vi "Get SMO Public API.vi"(8 "error in (no error)":errorcluster, 11 "Inst.Krohn-Hite-7008 in":refnum<class "Inst.Krohn-Hite-7008.lvclass">) -> (0 "error out":errorcluster, 2 "Commands":string[](array[string]), 3 "Inst.Krohn-Hite-7008 out":refnum<class "Inst.Krohn-Hite-7008.lvclass">)   [LabVIEW 2019, in "Inst.KH7008.lvlib" / "Inst.Krohn-Hite-7008.lvclass"]
uses:
  Inst.Krohn-Hite-7008.lvclass
  Typedefs/Inst.Krohn-Hite-7008.Commands--Enum.ctl
  d076ed97-22e4-4017-a7d1-2daba86b0ad5.vi
  5bb7ec78-ffd5-4b96-a1c9-711a63f6b5b1.vi
  <vilib>/Utility/Data Type/Get Type Information.vi
  <vilib>/Utility/Data Type/Get Numeric Information.vi
  <userlib>/_OpenG.lib/lvdata/lvdata.llb/Unwrap VVariant__ogtk.vi
  <userlib>/LevyLab/Instrument Framework/Instrument Types/Amplifier/Instrument.Amplifier.lvclass
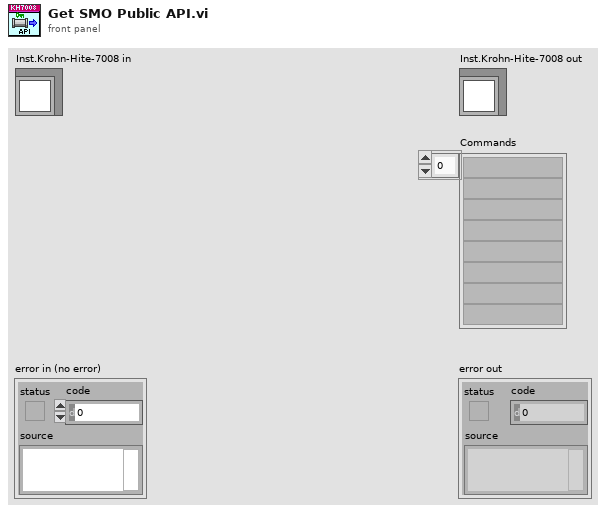
[diagram p1: front panel]
types:
  T1 = typedef "Inst.KH7008.lvlib/Inst.Krohn-Hite-7008.lvclass/Inst.Krohn-Hite-7008.Commands--Enum.ctl" = enum16{"getChannel", "getAllChannels", "setChannel", "setAllChannels"}
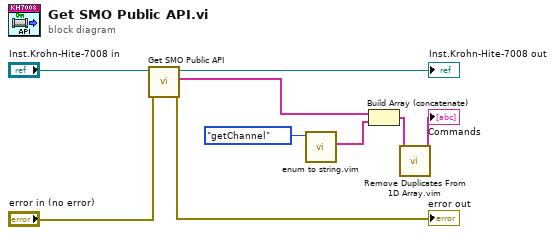
[diagram p0: block diagram]
diagram:
  n1 = call-parent "Get SMO Public API.vi"("error in (no error)"="error in (no error)", "Instrument.Amplifier in"="Inst.Krohn-Hite-7008 in") -> ("error out"=→"error out":errorcluster, "commands"=w9:string[], "Instrument.Amplifier out"=→"Inst.Krohn-Hite-7008 out":refnum<class "Inst.Krohn-Hite-7008.lvclass">)  [unwired: 7 in]
  n2 = call "enum to string.vim"("enum in"=Inst.Krohn-Hite-7008.Commands--Enum."getChannel" ("Commands")) -> ("strings out"=w5:string[])  [unwired: 9 in, 1 out]
  n3 = Build Array (concatenate)(w9, w5) -> (w2:string[])
  n4 = call "Remove Duplicates From 1D Array.vim"("array"=w2) -> ("array with duplicates removed"=→"Commands":string[])  [unwired: 10 in]
